vi "oa_TV Set Channel Info (Even Angle Output NChan).vi"(0 "seconds/revolution":cluster{dbl[]}[](array[cluster]), 1 "torisional vibration unit (RPM)":enum16{"RPM", "deg/s", "rad/s"}(ring), 5 "pulse positions":cluster{dbl[]}[](array[cluster]), 7 "pulse/revolution (1)":i32[](array[numeric]) min=1, 11 "error in (no error)":errorcluster, 12 "r0":dbl[](array[numeric]), 13 "dr":dbl[](array[numeric])) -> (4 "even-angle torsional vibration":cluster{"r0":dbl, "dr":dbl, "Y":dbl[]}[](array[cluster]), 6 "even-angle channel info":T3[](array[typedef]) {"channel info"."pregain" format="%.2f"; "channel info"."weighting filter" items=["Linear", "A-weighting", "B-weighting", "C-weighting", "ITU-R 468-4", "Dolby", "CCITT", "C-message", "Wb", "Wc", "Wd", "We", "Wf", "Wh", "Wj", "Wk", "Wm", "AES17 20 kHz lowpass", "AES17 40 kHz lowpass", "AES17 20 kHz highpass", "AES17 40 kHz highpass"]; "channel info"."dB reference" format="%^.1e"; "channel info"."engineering units" items=["custom..."=0, "V"=1, "A"=21, "C"=30, "pC"=31, "s"=32, "-"=29, "Pa"=2, "N"=20, "g"=3, "m/s^2"=4, "m/s"=5, "m"=6, "mm/s"=12, "mm"=13, "micron/s"=14, "micron"=15, "in/s^2"=7, "in/s"=8, "in"=9, "mil/s"=10, "mil"=11, "rad/s^2"=16, "rad/s"=17, "rad"=18, "deg/s^2"=26, "deg/s"=27, "deg"=28, "RPM"=22, "cycle/s^2"=23, "Hz"=24, "cycle"=25, "strain"=19]; "channel info"."sensor sensitivity" format="%#_5f"}, 8 "speed profiles":T2[](array[typedef]) {"speed [RPM]" format="%.2f"; "time [s]" format="%.2f"}, 10 "position info":T1[](array[typedef]), 14 "unit labels":string[](array[string]), 15 "error out":errorcluster)   [LabVIEW 2017, in "SoundVib_Torsional.lvlib"]
uses:
  <vilib>/addons/Sound and Vibration/Order Analysis/Torsional Vibration/SoundVib_Torsional.lvlib
  <vilib>/addons/_NISVFA/_Shared subVIs/Controls/svc_Resampled Channel Info.ctl
  <vilib>/addons/_NISVFA/_Shared subVIs/Controls/svc_Channel Info.ctl
  <vilib>/addons/_NISVFA/_Shared subVIs/Controls/svc_Engineering Units Text Ring.ctl
  <vilib>/addons/_NISVFA/_Shared subVIs/Controls/svc_Weighting Filter Text Ring.ctl
  <vilib>/addons/Sound and Vibration/Order Analysis/Tach Process/SubVIs/speed profile.ctl
  <vilib>/addons/Sound and Vibration/Order Analysis/Misc/OAT Position Info.ctl
  <vilib>/addons/Sound and Vibration/Order Analysis/Tach Process/SoundVib_TachProcess.lvlib
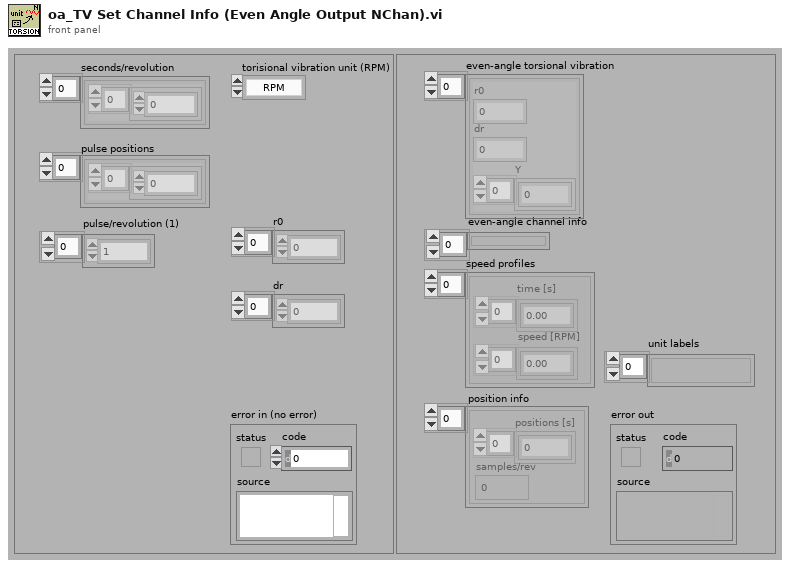
[diagram p1: front panel]
types:
  T1 = typedef "OAT Position Info.ctl" = cluster{"positions [s]":dbl[], "samples/rev":dbl}
  T2 = typedef "SoundVib_TachProcess.lvlib/speed profile.ctl" = cluster{"time [s]":dbl[], "speed [RPM]":dbl[]}
  T3 = typedef "svc_Resampled Channel Info.ctl" = cluster{"channel name":string, "description":string, " channel info":T4}
  T4 = typedef "svc_Channel Info.ctl" = cluster{"sensor sensitivity":dbl, "engineering units":T5, "dB reference":dbl, "custom label":string, "weighting filter":T6, "pregain":dbl}
  T5 = typedef "svc_Engineering Units Text Ring.ctl" = u16
  T6 = typedef "svc_Weighting Filter Text Ring.ctl" = u16
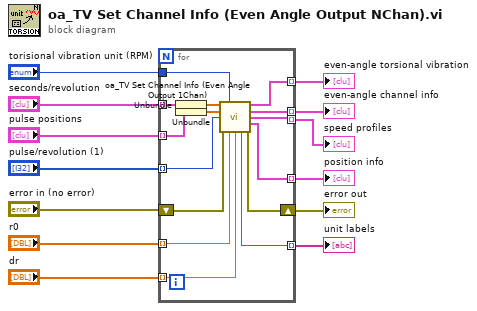
[diagram p0: block diagram]
diagram:
  n1 = for {
    shift-right: [w23] -> w12
    shift-left: "error in (no error)" -> [w24]
    tunnel: "seconds/revolution" -> [w27] mode=indexing
    tunnel: "torisional vibration unit (RPM)" -> [w20]
    tunnel: "r0" -> [w26] mode=indexing
    tunnel: "dr" -> [w25] mode=indexing
    tunnel: [w22] -> w8 mode=indexing
    tunnel: [w21] -> w7 mode=indexing
    tunnel: [w19] -> w5 mode=indexing
    tunnel: [w18] -> w2 mode=indexing
    tunnel: [w17] -> w1 mode=indexing
    tunnel: "pulse positions" -> [w16] mode=indexing
    tunnel: "pulse/revolution (1)" -> [w14] mode=indexing
    n2 = Unbundle(w27) -> (w28:dbl[])
    n3 = Unbundle(w16) -> (w15:dbl[])
    n4 = call <vilib>:"oa_TV Set Channel Info (Even Angle Output 1Chan).vi"("seconds/rev"=w28, "torisional vibration unit (RPM)"=w20, "pulse position"=w15, "pulse/revolution (1)"=w14, "error in (no error)"=w24, "r0"=w26, "dr"=w25) -> ("even-angle torsional vibration"=w22:cluster{"r0":dbl, "dr":dbl, "Y":dbl[]}, "even-angle channel info"=w21:T3, "speed profile"=w18:T2, "position info"=w17:T1, "unit label"=w19:string, "error out"=w23:errorcluster)  [unwired: 3 in]
  }
  "even-angle channel info" <- w7
  "error out" <- w12
  "even-angle torsional vibration" <- w8
  "unit labels" <- w5
  "speed profiles" <- w2
  "position info" <- w1
